vi "Overlord.vi"() -> ()   [LabVIEW 2014]
panel:
  out "Servo_Input":string
  in  "Arduino_IP":string
  out "Transport":string
  out "Winch PW":string
  out "Drum PW":string
  out "Scoop PW":string
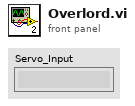
[diagram p1: front panel]
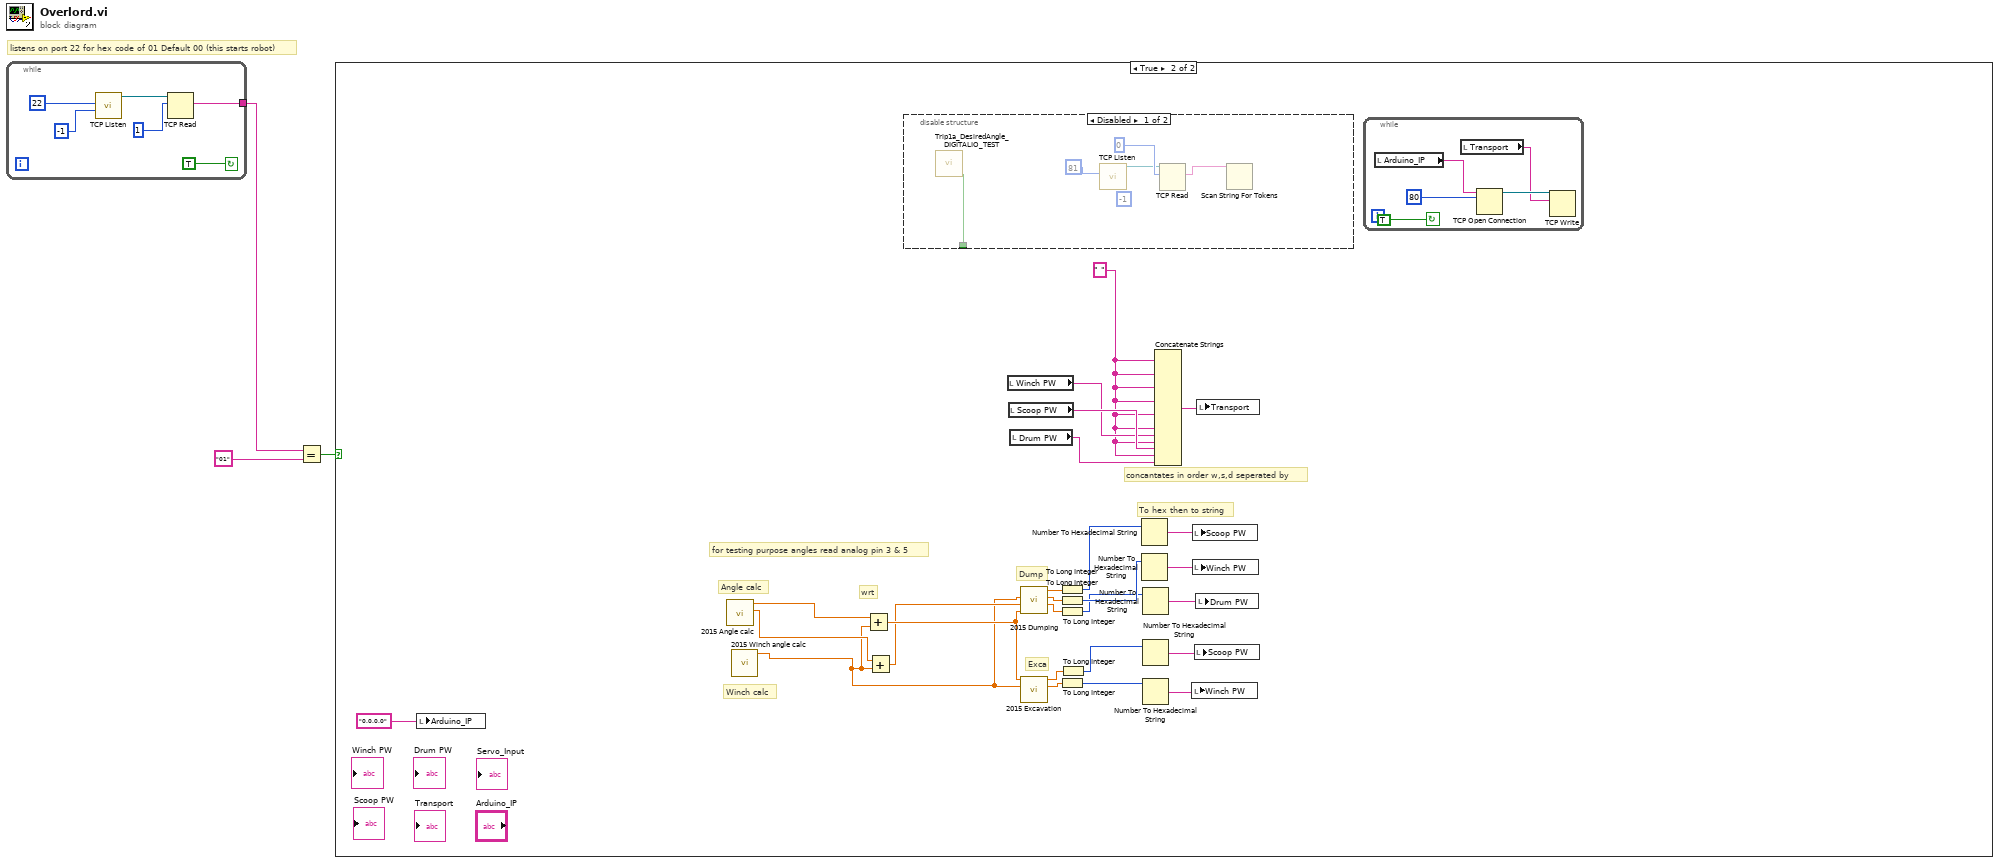
[diagram p0: block diagram]
diagram:
  # "listens on port 22 for hex code of 01 Default 00 (this starts robot)"
  n1 = while {
    tunnel: [w4] -> w2
    stop <- TRUE continue-if-true
    n2 = call <vilib>:"TCP Listen.vi"("timeout ms (wait forever: -1)"=-1, "port"=u16 22) -> ("connection ID"=w7:refnum<k5>)  [unwired: 5 in, 4 out]
    n3 = TCP Read(connection ID=w7, bytes to read=1) -> (data out=w4:string)  [unwired: 3 in, 2 out]
  }
  n4 = Equal?(x=w2, y="01") -> (x = y?=w3:bool)
  n5 = case shown="True" w3 {
    frame False {
    }
    frame True {
      w10 = " "
      # "To hex then to string"
      # "concantates in order w,s,d seperated by"
      # "Winch calc"
      # "wrt"
      # "Exca"
      # "Dump"
      # "for testing purpose angles read analog pin 3 & 5"
      # "Angle calc"
      n6 = local write "Arduino_IP"("0.0.0.0") -> ()
      n7 = call "2015 Angle calc.vi"() -> ("Drum angle"=w35:dbl, "Scoop angle"=w34:dbl)  [unwired: 10 in]
      n8 = call "2015 Winch angle calc.vi"() -> ("Winch angle"=w14:dbl)  [unwired: 11 in]
      n9 = Add(x=w34, y=w14) -> (x+y=w33:dbl)
      n10 = Add(x=w35, y=w14) -> (x+y=w32:dbl)
      n11 = disable-structure shown="Disabled" {
        disable-tunnel: [w40 _] -> _
        frame Disabled {
          (unwired) -1
          n12 = call "Trip1a_DesiredAngle_DIGITALIO_TEST.vi"() -> ("Commence Mining"=w40:bool)  [unwired: 11 in]
          n13 = call <vilib>:"TCP Listen.vi"("port"=u16 81) -> ("connection ID"=w37:refnum<k5>)  [unwired: 6 in, 4 out]
          n14 = TCP Read(connection ID=w37, bytes to read=0) -> (data out=w39:string)  [unwired: 3 in, 2 out]
          n15 = Scan String For Tokens(9:w39) -> ()  [unwired: 5 in, 4 out]
        }
        frame Enabled {
        }
      }
      n16 = local read "Winch PW"() -> (w11:string)
      n17 = local read "Scoop PW"() -> (w12:string)
      n18 = local read "Drum PW"() -> (w13:string)
      n19 = call "2015 Dumping.vi"("Scoop angle"=w33, "Drum angle"=w32, "Winch angle"=w14) -> ("Drum PW"=w28:dbl, "Winch PW"=w29:dbl, "Scoop PW"=w31:dbl)  [unwired: 4 in, 1 out]
      n20 = call "2015 Excavation.vi"("Winch angle"=w14, "Scoop angle"=w33) -> ("Winch PW"=w24:dbl, "Scoop PW"=w25:dbl)  [unwired: 8 in]
      n21 = To Long Integer(number=w31) -> (32bit integer=w30:i32)
      n22 = To Long Integer(number=w29) -> (32bit integer=w27:i32)
      n23 = To Long Integer(number=w28) -> (32bit integer=w26:i32)
      n24 = To Long Integer(number=w24) -> (32bit integer=w22:i32)
      n25 = To Long Integer(number=w25) -> (32bit integer=w23:i32)
      n26 = Number To Hexadecimal String(2:w30) -> (0:w21:string)  [unwired: 1 in]
      n27 = Number To Hexadecimal String(2:w27) -> (0:w20:string)  [unwired: 1 in]
      n28 = Number To Hexadecimal String(2:w26) -> (0:w19:string)  [unwired: 1 in]
      n29 = Number To Hexadecimal String(2:w23) -> (0:w18:string)  [unwired: 1 in]
      n30 = Number To Hexadecimal String(2:w22) -> (0:w17:string)  [unwired: 1 in]
      n31 = Concatenate Strings(w10, w10, w10, w10, w10, w10, w11, w10, w12, w10, w13) -> (w16:string)  [unwired: 6 in]
      n32 = local write "Winch PW"(w17) -> ()
      n33 = local write "Scoop PW"(w21) -> ()
      n34 = local write "Winch PW"(w20) -> ()
      n35 = local write "Scoop PW"(w18) -> ()
      n36 = local write "Drum PW"(w19) -> ()
      n37 = local write "Transport"(w16) -> ()
      n38 = while {
        stop <- TRUE continue-if-true
        n39 = local read "Arduino_IP"() -> (w43:string)
        n40 = local read "Transport"() -> (w44:string)
        n41 = TCP Open Connection(address=w43, remote port or service name=u16 80) -> (connection ID=w45:refnum<k5>)  [unwired: 3 in, 1 out]
        n42 = TCP Write(connection ID=w45, data in=w44) -> ()  [unwired: 2 in, 3 out]
      }
    }
  }
